vi "Logger.Variant.Read.vi"(8 "error in (no error)":errorcluster, 11 "VariantSets in":T2={"State"=enum."Init", "ImgPath"=path "", "WabcoPlate"="", "WabcoProduct"="", "ClientProduct"="", "ClientPlate"="", "TotalQuantity"=0, "OrderQuantity"=0, "Serial"=0, "Wabco"={"LaserJob"="", "AdditionalTxt"="037", "FactoryCode"="", "RevID"=0, "ForkID"=0, "FailuresLimit"=0, "GlobalCnt"=0, "ScannerProgram"=0, "SerialFormat"=enum."6 dig", "CoordA"={"X"=0.0, "Y"=0.0, "Angle"=0.0}, "CoordB"={"X"=0.0, "Y"=0.0, "Angle"=0.0}, "DMCconfig"=0}, "Client"={"LaserJob"="", "AdditionalTxt"="", "FactoryCode"="037", "RevID"=0, "ForkID"=0, "FailuresLimit"=0, "GlobalCnt"=0, "ScannerProgram"=0, "SerialFormat"=enum."6 dig", "CoordA"={"X"=0.0, "Y"=0.0, "Angle"=0.0}, "CoordB"={"X"=0.0, "Y"=0.0, "Angle"=0.0}, "DMCconfig"=0}}) -> (0 "error out":errorcluster, 1 "ClientPlateImg":picture, 2 "WabcoPlateImg":picture, 3 "VariantSets out":T2={"State"=enum."Init", "ImgPath"=path "", "WabcoPlate"="", "WabcoProduct"="", "ClientProduct"="", "ClientPlate"="", "TotalQuantity"=0, "OrderQuantity"=0, "Serial"=0, "Wabco"={"LaserJob"="", "AdditionalTxt"="037", "FactoryCode"="", "RevID"=0, "ForkID"=0, "FailuresLimit"=0, "GlobalCnt"=0, "ScannerProgram"=0, "SerialFormat"=enum."6 dig", "CoordA"={"X"=0.0, "Y"=0.0, "Angle"=0.0}, "CoordB"={"X"=0.0, "Y"=0.0, "Angle"=0.0}, "DMCconfig"=0}, "Client"={"LaserJob"="", "AdditionalTxt"="", "FactoryCode"="037", "RevID"=0, "ForkID"=0, "FailuresLimit"=0, "GlobalCnt"=0, "ScannerProgram"=0, "SerialFormat"=enum."6 dig", "CoordA"={"X"=0.0, "Y"=0.0, "Angle"=0.0}, "CoordB"={"X"=0.0, "Y"=0.0, "Angle"=0.0}, "DMCconfig"=0}}, 5 "OrdersTableIdx":i32, 7 "OrdersTable":string[][](array[string]))   [LabVIEW 2016]
uses:
  Logger.Variant.Sets.ctl
  Station/Station.Changeover.State.vi
  Station/Station.Plate.Properties.ctl
  Sequence/Sequence.Code.SerialFormat.ctl
  Drivers/V7310/LowLevel/V7310.Job.Sets.ctl
  Global/ApplicationGlobal.vi
  Drivers/V7310/LowLevel/V7310.Global.vi
panel:
  in  "SerialFormat":T1
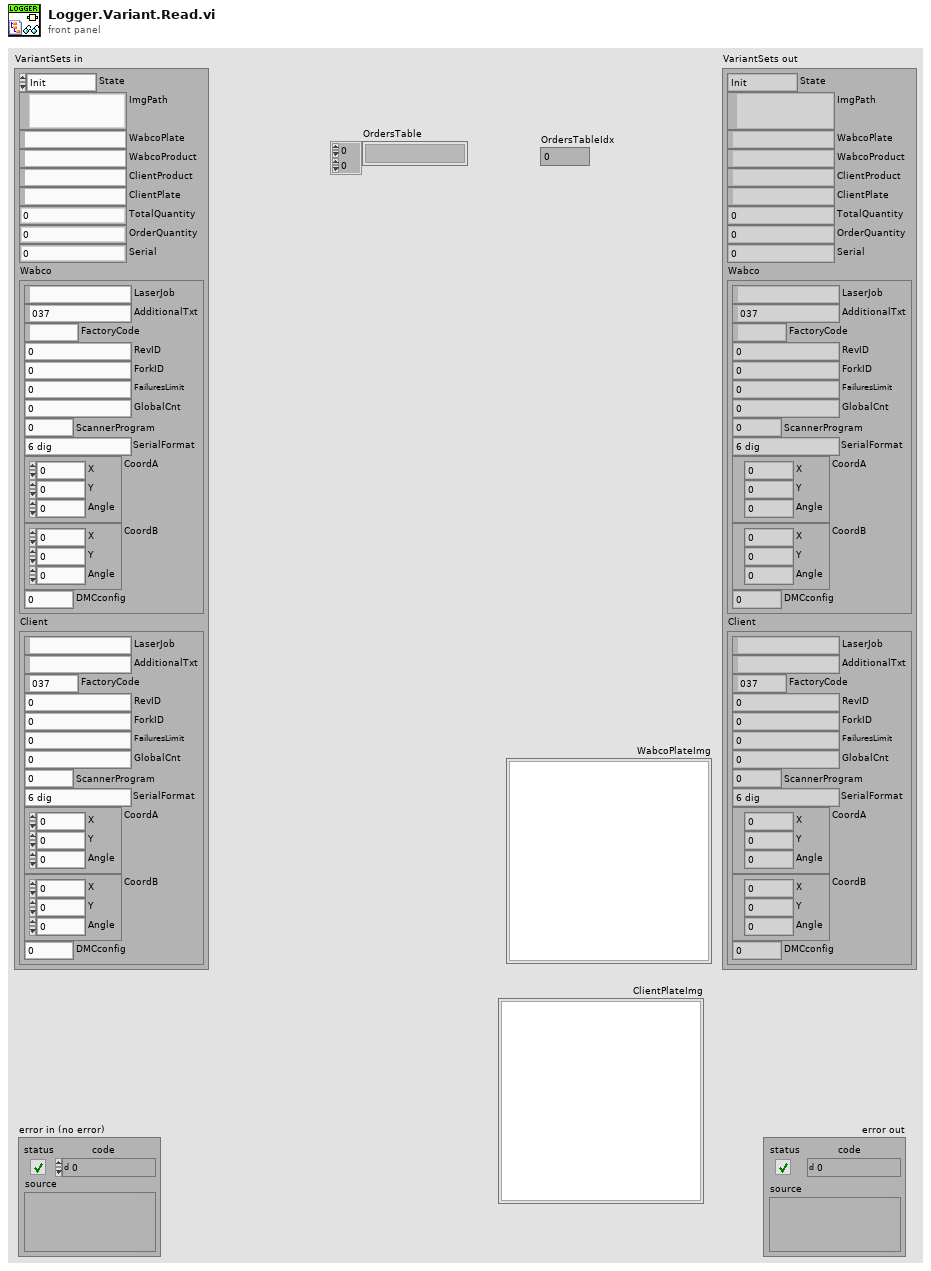
[diagram p1: front panel]
types:
  T1 = typedef "Sequence.Code.SerialFormat.ctl" = enum8{"", "6 dig", "7 dig"}
  T2 = typedef "Logger.Variant.Sets.ctl" = cluster{"State":T3, "ImgPath":path, "WabcoPlate":string, "WabcoProduct":string, "ClientProduct":string, "ClientPlate":string, "TotalQuantity":u16, "OrderQuantity":u16, "Serial":i32, "Wabco":T4, "Client":T4}
  T3 = typedef "Station.Changeover.State.vi" = enum16{"Init", "Scaning", "NOK", "Wait for ack", "Ready"}
  T4 = typedef "Station.Plate.Properties.ctl" = cluster{"LaserJob":string, "AdditionalTxt":string, "FactoryCode":string, "RevID":u8, "ForkID":u8, "FailuresLimit":u16, "GlobalCnt":i32, "ScannerProgram":u8, "SerialFormat":T1, "CoordA":T5, "CoordB":T5, "DMCconfig":i32}
  T5 = typedef "V7310.Job.Sets.ctl" = cluster{"X":dbl, "Y":dbl, "Angle":dbl}
  T6 = cluster{"WabcoPlate":string, "WabcoProduct":string, "ClientProduct":string, "ClientPlate":string}
  T7 = typedef "imagedata.ctl" = cluster{"image type":i32, "image depth":i32, "image":u8[], "mask":u8[], "colors":u32[], "Rectangle":cluster{"left":i16, "top":i16, "right":i16, "bottom":i16}}
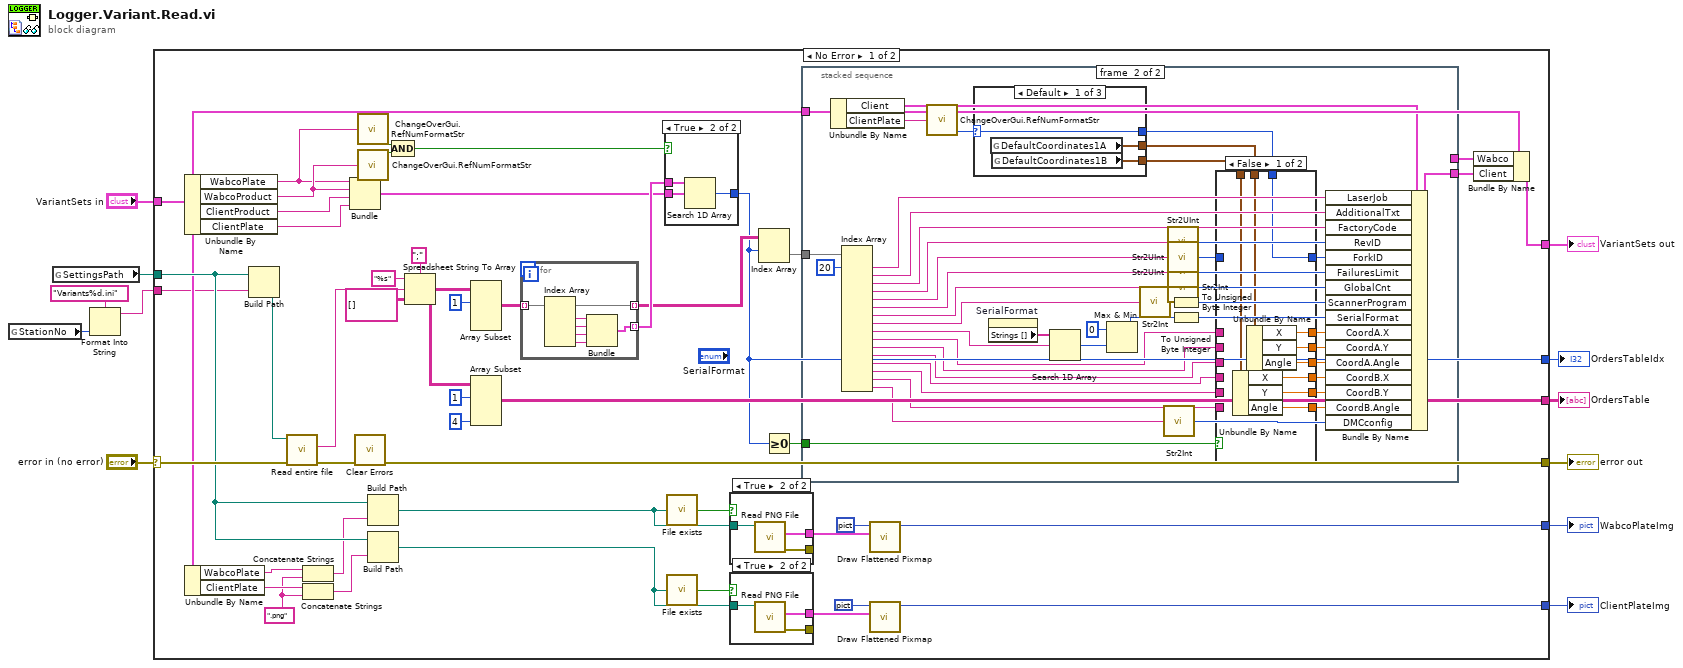
[diagram p0: block diagram]
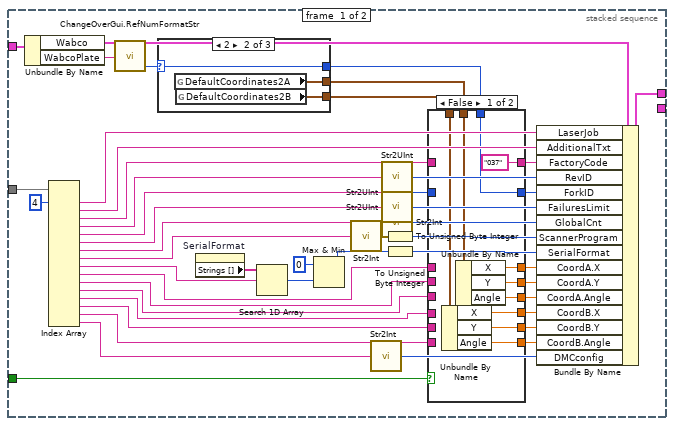
[diagram p2: hidden frame]
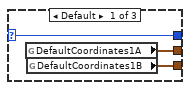
[diagram p3: hidden frame]
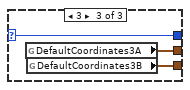
[diagram p4: hidden frame]
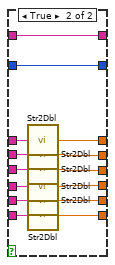
[diagram p5: hidden frame]
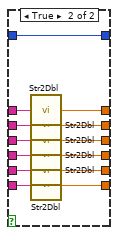
[diagram p6: hidden frame]
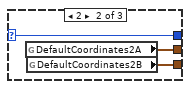
[diagram p7: hidden frame]
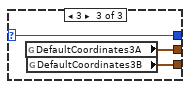
[diagram p8: hidden frame]
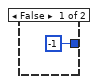
[diagram p9: hidden frame]
diagram:
  n1 = global read "ApplicationGlobal.vi" "StationNo"() -> (w2:i32)
  n2 = global read "ApplicationGlobal.vi" "SettingsPath"() -> (w10:path)
  n3 = Format Into String(format string="Variants%d.ini", w2) -> (resulting string=w1:string)  [unwired: 2 in, 1 out]
  n4 = case shown="No Error" "error in (no error)" {
    selector: "error in (no error)" -> [w59 w234]
    tunnel: [w28 w234] -> w11
    tunnel: w10 -> [w50 _]
    tunnel: [w24 _] -> w8
    tunnel: [w60 _] -> w9
    tunnel: "VariantSets in" -> [w16 _]
    tunnel: [w39 _] -> w6
    tunnel: [w17 _] -> w5
    tunnel: [w15 _] -> w4
    tunnel: w1 -> [w13 _]
    frame No Error {
      w46 = ".png" ("string")
      n5 = Unbundle By Name(w16) -> ("WabcoPlate"=w30:string, "WabcoProduct"=w31:string, "ClientProduct"=w37:string, "ClientPlate"=w21:string)
      n6 = Unbundle By Name(w16) -> ("WabcoPlate"=w47:string, "ClientPlate"=w49:string)
      n7 = Build Path(base path=w50, name or relative path=w13) -> (appended path=w55:path)
      n8 = call "Read entire file.vi"("error in"=w59, "file"=w55) -> ("error out"=w34:errorcluster, "contents"=w54:string)  [unwired: 4 in]
      n9 = Concatenate Strings(w47, w46) -> (w45:string)
      n10 = Concatenate Strings(w49, w46) -> (w48:string)
      n11 = Bundle("WabcoPlate"=w30, "WabcoProduct"=w31, "ClientProduct"=w37, "ClientPlate"=w21) -> (w35:T6)  [unwired: 1 in]
      n12 = call <vilib>:"Clear Errors.vi"("error in (no error)"=w34) -> ("error out"=w28:errorcluster)  [unwired: 5 in, 1 out]
      n13 = call "ChangeOverGui.RefNumFormatStr.vi"("RefNum in"=w30) -> ("RefNum format ok?"=w33:bool)  [unwired: 2 out]
      n14 = call "ChangeOverGui.RefNumFormatStr.vi"("RefNum in"=w31) -> ("RefNum format ok?"=w32:bool)  [unwired: 2 out]
      n15 = Build Path(base path=w50, name or relative path=w45) -> (appended path=w44:path)
      n16 = Build Path(base path=w50, name or relative path=w48) -> (appended path=w40:path)
      n17 = Compound Arithmetic op=AND(w33, w32) -> (w29:bool)
      n18 = Spreadsheet String To Array(delimiter (Tab)=";", format string="%s", spreadsheet string=w54, array type (2D Dbl)=string[][] []) -> (array=w20:string[][])
      n19 = Array Subset(array=w20, index (row)=1 ("index")) -> (w27:string[][])  [unwired: 3 in]
      n20 = Array Subset(array=w20, index (row)=1 ("index"), length (col)=4 ("length")) -> (w17:string[][])  [unwired: 2 in]
      n21 = for {
        tunnel: w27 -> [w219] mode=indexing
        tunnel: [w220] -> w36 mode=indexing
        tunnel: [w219] -> w26 mode=indexing
        n22 = Index Array(array=w219) -> (element #1=w223:string, element #2=w222:string, element #3=w221:string, element #4=w218:string)  [unwired: 4 in]
        n23 = Bundle(w223, w222, w221, w218) -> (w220:cluster{string, string, string, string})  [unwired: 1 in]
      }
      n24 = case shown="True" w29 {
        tunnel: w36 -> [_ w227]
        tunnel: w35 -> [_ w226]
        tunnel: [-1 ("index of element") w225] -> w15
        frame False {
        }
        frame True {
          n25 = Search 1D Array(1D array=w227, element=w226) -> (index of element=w225:i32)  [unwired: 1 in]
        }
      }
      n26 = call "File exists.vi"("file path"=w44) -> ("exists?"=w58:bool)  [unwired: 4 in]
      n27 = call "File exists.vi"("file path"=w40) -> ("exists?"=w41:bool)  [unwired: 4 in]
      n28 = case shown="True" w58 {
        tunnel: w44 -> [_ w233]
        tunnel: [_ w232] -> w56
        tunnel: [_ w231] -> _
        frame False {
        }
        frame True {
          n29 = call <vilib>:"Read PNG File.vi"("path to PNG file"=w233) -> ("error out"=w231:errorcluster, "image data"=w232:T7)  [unwired: 8 in, 1 out]
        }
      }
      n30 = case shown="True" w41 {
        tunnel: w40 -> [_ w230]
        tunnel: [_ w229] -> w43
        tunnel: [_ w228] -> _
        frame False {
        }
        frame True {
          n31 = call <vilib>:"Read PNG File.vi"("path to PNG file"=w230) -> ("error out"=w228:errorcluster, "image data"=w229:T7)  [unwired: 8 in, 1 out]
        }
      }
      n32 = Index Array(array=w26, index (row)=w15) -> (element=w25:string[])  [unwired: 1 in]
      n33 = Greater Or Equal To 0?(x=w15) -> (x >= 0?=w14:bool)
      n34 = stacked-sequence {
        tunnel: w25 -> [w105 w184]
        tunnel: w16 -> [w77 w166]
        tunnel: [w103 _] -> w23
        tunnel: [_ w167] -> w22
        tunnel: w14 -> [w76 w163]
        frame #0 {
          n35 = Unbundle By Name(w77) -> ("Wabco"=w107:T4, "WabcoPlate"=w75:string)
          n36 = Index Array(array=w105, index #1=4 ("index")) -> (element #1=w104:string, element #2=w102:string, element #3=w71:string, element #4=w100:string, element #5=w63:string, element #6=w98:string, element #7=w96:string, element #8=w61:string, element #9=w84:string, element #10=w83:string, element #11=w82:string, element #12=w81:string, element #13=w80:string, element #14=w79:string, element #15=w78:string, element #16=w67:string)  [unwired: 15 in]
          n37 = call "ChangeOverGui.RefNumFormatStr.vi"("RefNum in"=w75) -> ("Idx"=w74:i32)  [unwired: 2 out]
          n38 = case shown="2" w74 {
            selector: w74 -> [w108 w111 w114]
            tunnel: [w110 w113 w116] -> w73
            tunnel: [w109 w112 w115] -> w72
            tunnel: [w108 w111 w114] -> w69
            frame Default {
              n39 = global read "V7310.Global.vi" "DefaultCoordinates1A"() -> (w110:T5)
              n40 = global read "V7310.Global.vi" "DefaultCoordinates1B"() -> (w109:T5)
            }
            frame 2 {
              n41 = global read "V7310.Global.vi" "DefaultCoordinates2A"() -> (w113:T5)
              n42 = global read "V7310.Global.vi" "DefaultCoordinates2B"() -> (w112:T5)
            }
            frame 3 {
              n43 = global read "V7310.Global.vi" "DefaultCoordinates3A"() -> (w116:T5)
              n44 = global read "V7310.Global.vi" "DefaultCoordinates3B"() -> (w115:T5)
            }
          }
          n45 = property on="SerialFormat" class="Enum (strict)"() -> ("Strings []"=w95:string[])  [unwired: 2 in, 2 out]
          n46 = Search 1D Array(1D array=w95, element=w84) -> (index of element=w94:i32)  [unwired: 1 in]
          n47 = Max & Min(x=0, y=w94) -> (max(x,y)=w91:i32)  [unwired: 1 out]
          n48 = call "Str2Int.vi"("string"=w61) -> ("Numeric"=w64:i32)
          n49 = call "Str2Int.vi"("string"=w67) -> ("Numeric"=w66:i32)
          n50 = call "Str2UInt.vi"("string"=w100) -> ("Numeric"=w101:u32)
          n51 = call "Str2UInt.vi"("string"=w63) -> ("Numeric"=w62:u32)
          n52 = call "Str2UInt.vi"("string"=w98) -> ("Numeric"=w99:u32)
          n53 = call "Str2Int.vi"("string"=w96) -> ("Numeric"=w97:i32)
          n54 = To Unsigned Byte Integer(number=w64) -> (unsigned 8bit integer=w65:u8)
          n55 = To Unsigned Byte Integer(number=w91) -> (unsigned 8bit integer=w92:u8)
          n56 = case shown="False" w76 {
            tunnel: [w125 w140] -> w90
            tunnel: [w124 w139] -> w89
            tunnel: [w123 w138] -> w88
            tunnel: [w121 w137] -> w87
            tunnel: [w120 w136] -> w86
            tunnel: [w119 w135] -> w85
            tunnel: w83 -> [_ w134]
            tunnel: w82 -> [_ w133]
            tunnel: w81 -> [_ w132]
            tunnel: w80 -> [_ w131]
            tunnel: w79 -> [_ w130]
            tunnel: w78 -> [_ w129]
            tunnel: w73 -> [w126 _]
            tunnel: w72 -> [w122 _]
            tunnel: w71 -> [_ w128]
            tunnel: ["037" w128] -> w70
            tunnel: w69 -> [w117 _]
            tunnel: [w117 w127] -> w68
            tunnel: w62 -> [_ w127]
            frame False {
              n57 = Unbundle By Name(w122) -> ("X"=w121:dbl, "Y"=w120:dbl, "Angle"=w119:dbl)
              n58 = Unbundle By Name(w126) -> ("X"=w125:dbl, "Y"=w124:dbl, "Angle"=w123:dbl)
            }
            frame True {
              n59 = call "Str2Dbl.vi"("string"=w134) -> ("Numeric"=w140:dbl)
              n60 = call "Str2Dbl.vi"("string"=w133) -> ("Numeric"=w139:dbl)
              n61 = call "Str2Dbl.vi"("string"=w132) -> ("Numeric"=w138:dbl)
              n62 = call "Str2Dbl.vi"("string"=w131) -> ("Numeric"=w137:dbl)
              n63 = call "Str2Dbl.vi"("string"=w130) -> ("Numeric"=w136:dbl)
              n64 = call "Str2Dbl.vi"("string"=w129) -> ("Numeric"=w135:dbl)
            }
          }
          n65 = Bundle By Name(cluster=w107, "LaserJob"=w104, "AdditionalTxt"=w102, "FactoryCode"=w70, "RevID"=w101, "ForkID"=w68, "FailuresLimit"=w99, "GlobalCnt"=w97, "ScannerProgram"=w65, "SerialFormat"=w92, "CoordA.X"=w90, "CoordA.Y"=w89, "CoordA.Angle"=w88, "CoordB.X"=w87, "CoordB.Y"=w86, "CoordB.Angle"=w85, "DMCconfig"=w66) -> (w103:T4)
        }
        frame #1 {
          n66 = Unbundle By Name(w166) -> ("Client"=w186:T4, "ClientPlate"=w164:string)
          n67 = Index Array(array=w184, index #1=20 ("index")) -> (element #1=w183:string, element #2=w182:string, element #3=w181:string, element #4=w179:string, element #5=w178:string, element #6=w176:string, element #7=w174:string, element #8=w141:string, element #9=w168:string, element #10=w160:string, element #11=w159:string, element #12=w158:string, element #13=w161:string, element #14=w162:string, element #15=w157:string, element #16=w145:string)  [unwired: 15 in]
          n68 = call "ChangeOverGui.RefNumFormatStr.vi"("RefNum in"=w164) -> ("Idx"=w165:i32)  [unwired: 2 out]
          n69 = case shown="Default" w165 {
            selector: w165 -> [w209 w212 w215]
            tunnel: [w211 w214 w217] -> w156
            tunnel: [w210 w213 w216] -> w155
            tunnel: [w209 w212 w215] -> w147
            frame Default {
              n70 = global read "V7310.Global.vi" "DefaultCoordinates1A"() -> (w211:T5)
              n71 = global read "V7310.Global.vi" "DefaultCoordinates1B"() -> (w210:T5)
            }
            frame 2 {
              n72 = global read "V7310.Global.vi" "DefaultCoordinates2A"() -> (w214:T5)
              n73 = global read "V7310.Global.vi" "DefaultCoordinates2B"() -> (w213:T5)
            }
            frame 3 {
              n74 = global read "V7310.Global.vi" "DefaultCoordinates3A"() -> (w217:T5)
              n75 = global read "V7310.Global.vi" "DefaultCoordinates3B"() -> (w216:T5)
            }
          }
          n76 = property on="SerialFormat" class="Enum (strict)"() -> ("Strings []"=w173:string[])  [unwired: 2 in, 2 out]
          n77 = Search 1D Array(1D array=w173, element=w168) -> (index of element=w172:i32)  [unwired: 1 in]
          n78 = Max & Min(x=0, y=w172) -> (max(x,y)=w169:i32)  [unwired: 1 out]
          n79 = call "Str2Int.vi"("string"=w141) -> ("Numeric"=w142:i32)
          n80 = call "Str2Int.vi"("string"=w145) -> ("Numeric"=w144:i32)
          n81 = call "Str2UInt.vi"("string"=w179) -> ("Numeric"=w180:u32)
          n82 = call "Str2UInt.vi"("string"=w178) -> ("Numeric"=w146:u32)
          n83 = call "Str2UInt.vi"("string"=w176) -> ("Numeric"=w177:u32)
          n84 = call "Str2Int.vi"("string"=w174) -> ("Numeric"=w175:i32)
          n85 = To Unsigned Byte Integer(number=w142) -> (unsigned 8bit integer=w143:u8)
          n86 = To Unsigned Byte Integer(number=w169) -> (unsigned 8bit integer=w170:u8)
          n87 = case shown="False" w163 {
            tunnel: [w194 w208] -> w154
            tunnel: [w193 w207] -> w153
            tunnel: [w192 w206] -> w152
            tunnel: [w190 w205] -> w151
            tunnel: [w189 w204] -> w150
            tunnel: [w188 w203] -> w149
            tunnel: w156 -> [w195 _]
            tunnel: w155 -> [w191 _]
            tunnel: w162 -> [_ w202]
            tunnel: w161 -> [_ w201]
            tunnel: w160 -> [_ w200]
            tunnel: w159 -> [_ w199]
            tunnel: w158 -> [_ w198]
            tunnel: w157 -> [_ w197]
            tunnel: [w187 w196] -> w148
            tunnel: w147 -> [w187 _]
            tunnel: w146 -> [_ w196]
            frame False {
              n88 = Unbundle By Name(w191) -> ("X"=w190:dbl, "Y"=w189:dbl, "Angle"=w188:dbl)
              n89 = Unbundle By Name(w195) -> ("X"=w194:dbl, "Y"=w193:dbl, "Angle"=w192:dbl)
            }
            frame True {
              n90 = call "Str2Dbl.vi"("string"=w200) -> ("Numeric"=w208:dbl)
              n91 = call "Str2Dbl.vi"("string"=w199) -> ("Numeric"=w207:dbl)
              n92 = call "Str2Dbl.vi"("string"=w198) -> ("Numeric"=w206:dbl)
              n93 = call "Str2Dbl.vi"("string"=w201) -> ("Numeric"=w205:dbl)
              n94 = call "Str2Dbl.vi"("string"=w202) -> ("Numeric"=w204:dbl)
              n95 = call "Str2Dbl.vi"("string"=w197) -> ("Numeric"=w203:dbl)
            }
          }
          n96 = Bundle By Name(cluster=w186, "LaserJob"=w183, "AdditionalTxt"=w182, "FactoryCode"=w181, "RevID"=w180, "ForkID"=w148, "FailuresLimit"=w177, "GlobalCnt"=w175, "ScannerProgram"=w143, "SerialFormat"=w170, "CoordA.X"=w154, "CoordA.Y"=w153, "CoordA.Angle"=w152, "CoordB.X"=w151, "CoordB.Y"=w150, "CoordB.Angle"=w149, "DMCconfig"=w144) -> (w167:T4)
        }
      }
      n97 = call <vilib>:"Draw Flattened Pixmap.vi"("image data"=w56, "picture"=picture data[5B]) -> ("new picture"=w60:picture)  [unwired: 7 in]
      n98 = call <vilib>:"Draw Flattened Pixmap.vi"("image data"=w43, "picture"=picture data[5B]) -> ("new picture"=w39:picture)  [unwired: 7 in]
      n99 = Bundle By Name(cluster=w16, "Wabco"=w23, "Client"=w22) -> (w24:T2)
    }
    frame Error {
    }
  }
  "error out" <- w11
  "WabcoPlateImg" <- w9
  "VariantSets out" <- w8
  "ClientPlateImg" <- w6
  "OrdersTable" <- w5
  "OrdersTableIdx" <- w4
